vi "Configure from JSON.vi"(8 "error in (no error)":errorcluster, 9 "JSON Data":string, 10 "Version":u32, 11 "Device in":refnum<class "Device.lvclass">) -> (0 "error out":errorcluster, 3 "Device out":refnum<class "Device.lvclass">)   [LabVIEW 2015, in "IBEX Device.lvlib" / "Device.lvclass"]
doc: "Provides a means of configuring the device based on JSON data."
uses:
  Device.lvclass
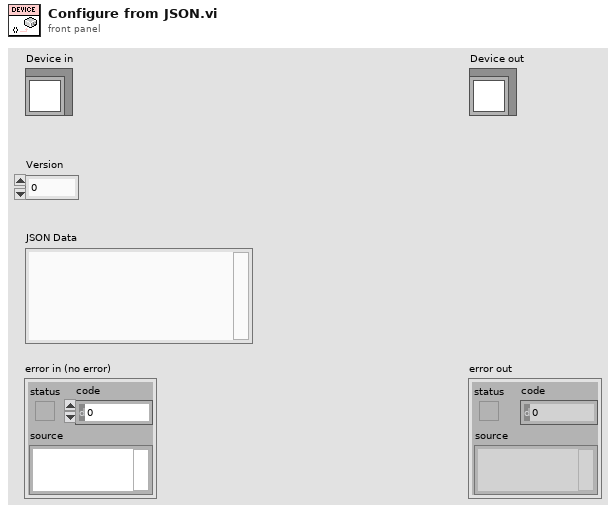
[diagram p1: front panel]
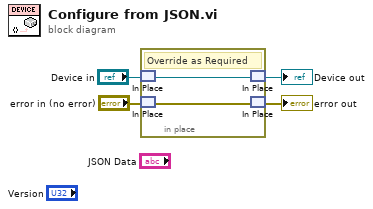
[diagram p0: block diagram]
diagram:
  n1 = in-place {
    # "Override as Required"
    n2 = in-place-match #1("Device in") -> (w6:refnum<class "Device.lvclass">)
    n3 = in-place-match #2("error in (no error)") -> (w5:errorcluster)
    n4 = in-place-match #1(w6) -> (→"Device out":refnum<class "Device.lvclass">)
    n5 = in-place-match #2(w5) -> (→"error out":errorcluster)
  }
